vi "VIP to Package URL.vi"(7 "Include Repository?":bool, 11 "VIP Information":T1) -> (3 "VIP Package URL":string)   [LabVIEW 2017, in "VIP SBOM Support.lvlib"]
doc: "Converts VIP information into a pURL package URL specification format."
uses:
  VIP SBOM Support.lvlib
  <vilib>/JKI/VIPM API/command-line/support/Library Contents Cluster_vipm_api.ctl
  <vilib>/wsapi/NI_WebServices.lvlib
  <vilib>/JKI/VIPM API/VIPM API_vipm_api.lvlib
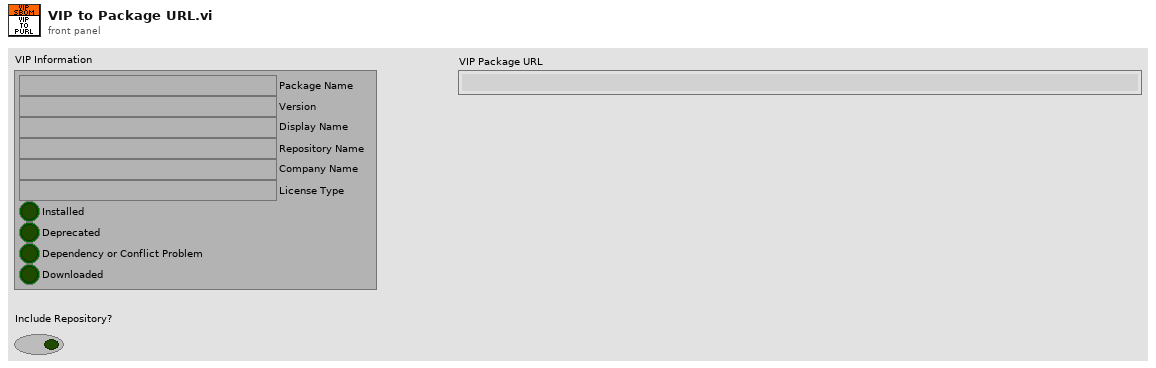
[diagram p1: front panel]
types:
  T1 = typedef "VIPM API_vipm_api.lvlib/Library Contents Cluster_vipm_api.ctl" = cluster{"Package Name":string, "Version":string, "Display Name":string, "Repository Name":string, "Company Name":string, "License Type":string, "Installed":bool, "Deprecated":bool, "Dependency or Conflict Problem":bool, "Downloaded":bool}
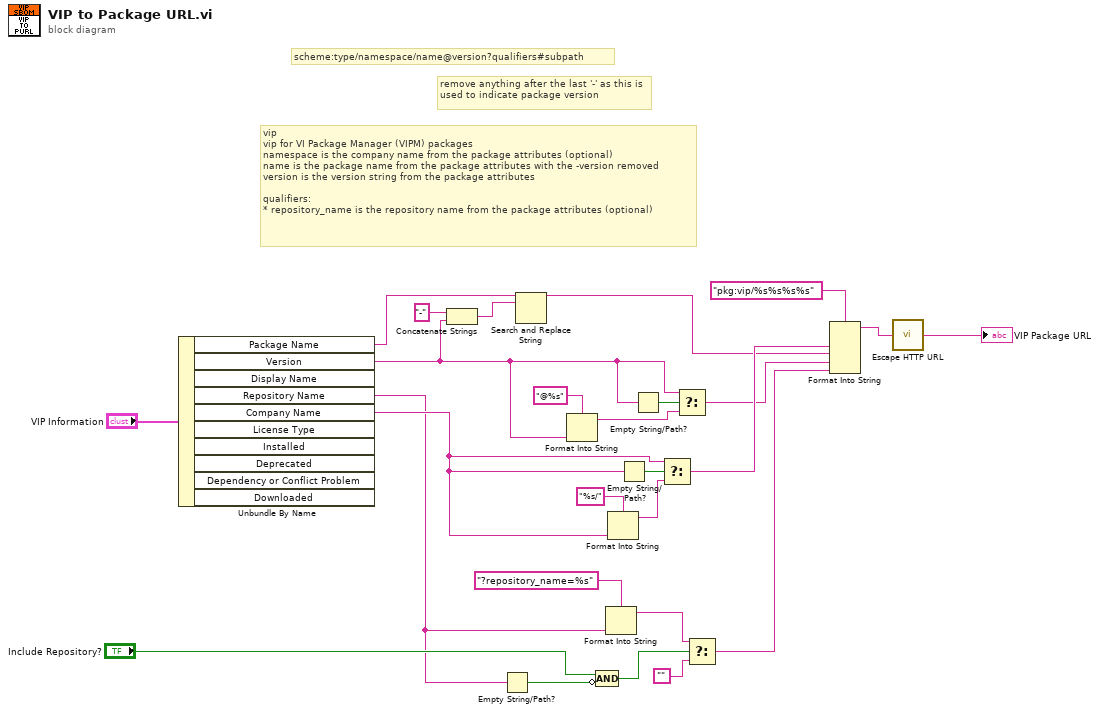
[diagram p0: block diagram]
diagram:
  # "vip\nvip for VI Package Manager (VIPM) packages\nnamespace is the company name from the package attributes (optional)\nname is the package name from the package attributes with the -version removed\nversion is the version string from the package attributes\n\nqualifiers:\n* repository_name is the repository name from the package attributes (optional)"
  # "remove anything after the last '-' as this is used to indicate package version"
  # "scheme:type/namespace/name@version?qualifiers#subpath"
  n1 = Unbundle By Name("VIP Information") -> ("Package Name"=w5:string, "Version"=w3:string, "Repository Name"=w10:string, "Company Name"=w20:string)  [unwired: 6 out]
  n2 = Concatenate Strings("-" ("string"), w3) -> (w2:string)
  n3 = Empty String/Path?(string/path=w10) -> (empty?=w11:bool)
  n4 = Search and Replace String(input string=w5, search string=w2) -> (result string=w1:string)  [unwired: 6 in, 3 out]
  n5 = Format Into String(format string="@%s", w3) -> (resulting string=w8:string)  [unwired: 2 in, 1 out]
  n6 = Compound Arithmetic op=AND("Include Repository?", invert w11) -> (w12:bool)
  n7 = Format Into String(format string="?repository_name=%s", w10) -> (resulting string=w17:string)  [unwired: 2 in, 1 out]
  n8 = Format Into String(format string="%s/", w20) -> (resulting string=w19:string)  [unwired: 2 in, 1 out]
  n9 = Empty String/Path?(string/path=w20) -> (empty?=w22:bool)
  n10 = Empty String/Path?(string/path=w3) -> (empty?=w6:bool)
  n11 = Select(t=w20, s=w22, f=w19) -> (s? t:f=w21:string)
  n12 = Select(t=w3, s=w6, f=w8) -> (s? t:f=w7:string)
  n13 = Select(t=w17, s=w12, f="") -> (s? t:f=w15:string)
  n14 = Format Into String(format string="pkg:vip/%s%s%s%s", w21, w1, w7, w15) -> (resulting string=w24:string)  [unwired: 2 in, 1 out]
  n15 = call <vilib>:"Escape HTTP URL.vi"("unescaped string in"=w24) -> ("escaped string out"=→"VIP Package URL":string)
